vi "Data Stream Control.vi"(4 "ready for input?":bool=TRUE caption="ready for input? (true)", 6 "force error":bool caption="force error (false)", 7 "stream.num samples 0":u64, 9 "data valid":bool=TRUE caption="data valid (true)", 10 "element count":u16=1 caption="element count (1)", 11 "stream.request state 0":T1) -> (0 "request data":bool, 1 "send data":bool, 2 "stream.state 0":T1, 3 "stream.samples transferred 0":u64, 5 "stream.metadata 0":u64)   [LabVIEW 2015, in "niInstr Streaming v1 FPGA.lvlib"]
doc: "<B>General</B>\n\nThis VI gates the assertion of <B>send data</B> with a state machine controller. This enables the control and monitoring of finite and continuous streams of data.\n\n<B>Signals</B>\n\nThe stream is controlled by the <B>stream.request state</B> and <B>stream.num samples</B> inputs. The stream is monitored by the <B>stream.state</B> and <B>stream.samples transferred</B> outputs. In addition, <b>stream.metadata</b> is available for publishing details about the form/function of the stream.\n\nWhen <B>data valid</B> is True, and <B>ready for input?</B> is True, the Data Stream Control will assert <B>send data</B> until the transfer completes.\n\nWhen <B>data valid</B> is True, but <B>ready for input?</B> is False, the stream stops asserting <B>send data</B> and enters the \"Error\" state.\n\nWhen <B>force error</B> is True, the stream is forced into the Error state. This allows user logic to monitor for fatal conditions and stop the stream.\n\n<B>stream.samples transferred</B> is updated after the \"data valid\" clock cycle that increments it. This enables this output to have an easier time meeting the timed loop deadline, as well as enables it to be directly wired up as an indexing input to a write memory element.\n\n<B>request data</b> informs upstream nodes that the Data Stream Control is requesting data delivery in the next clock cycle.\n\nNote, however, that the Data Stream Control does not provide caching. Typical users wishing to avoid overflows should directly connect the \"ready for input?\" terminal to upstream data, as well as to the Data Stream Control.\n\n<b>ready for data?</b> informs the Data Stream Control that the downstream node is ready to accept data.\n\n<B>Detailed Operation</B>\n\nThe state machine has two fundamental modes of transfer: \"Finite\" and \"Continuous.\"\n\nIn Finite mode, the state machine will count <B>stream.num samples</B> in increments of <B>element count</B>. When the count is equal to or exceeds <B>stream.num samples</B>, it prevents the assertion of <B>send data</B> and enters the Done state. In the \"Done\" state the samples transferred continues to be reported until the user requests that the state machine return to \"Idle.\"\n\nIn Continuous mode, the state machine will behave identically to Finite mode, but will continously transfer samples instead of counting them.\n\n<b>States</b>\n\nThere are seven potential states for a stream defined by the Stream State.ctl typedef. All commanded states should be monitored from the controlling loop if it is important to ensure that the state is actually entered. The <B>stream.request state</B> commands the stream into a state, and <B>stream.state</B> reflects the current actual state.\n\n\nIdle - when the stream is ready to enter into an active state, it is in the Idle state. While it can be commanded directly to Idle from any state (other than Not Ready), it is advisable to do so with caution as samples abandoned in transfers may still need to be manually cleared out. It is generally safe to go directly from \"Done\" to \"Idle,\" and it is generally safe to request a transition from \"Not Ready\" to \"Idle.\" Other states may require further clean-up such as stopping/starting FIFOs or resetting other code under the command of the stream. Consider using \"Cancel\" instead (such as through the \"Stop Stream.vi\" in the host environment).\n\nWhile in Idle, <B>stream.samples transferred</B> is reset to 0. \n\nFinite Transfer - Execute a transfer for the requested number of samples. <B>data valid</B> is passed through to <B>send data</B> until the stream terminates. Upon an orderly completion, this VI will automatically enter the Done state. If a stream overflows because <B>data valid</B> is True, but <B>ready for input?</B> is False, the stream stops asserting <B>send data</B> and enters the \"Error\" state.\n\nContinuous - Execute a transfer indefinitely. This state operates identically to the Finite Transfer state, but without regard to the <B>stream.num samples</B> input.\n\nDone - In an orderly termination of a finite stream, the stream should end up here. At this point, <B>stream.samples transferred</B> accurately reflects the terminal state of the transfer. The \"Done\" state should be exited by requesting \"Idle.\" \"Cancel\" or further active transfer modes (Finite or Continuous) will be ignored. This allows the host to distinguish between streams that are prematurely terminated (thus potentially requiring a flush of abandoned data) and ones that completed naturally.\n\nError - If the stream detects an unplanned interruption of the data, it enters the Error state. The error state is normally considered a fatal state, although one may enter it purposefully (such as at the end of a long, Continuous mode Host to Target transfer). The only way to exit the Error state is to command the Data Stream Control back to Idle, or reset the FPGA VI. When commanded to Idle, the Data Stream Control advances first to \"Not Ready.\" See that state for more information.\n\nNot Ready - In this state, the FPGA remains Not Ready until the \"ready for input?\" parameter becomes true. This prevents starting a transfer in an obviously invalid state, and allows host control to wait until the \"not ready\" state is removed (such as by clearing out a FIFO under the streaming API's control). Although unusual to command the stream into this state, a client may use the features of this state to avoid going to idle until the FPGA indicates readiness.\n\nCancel - this state is indistinguishable from \"Done,\" but allows the controlling VI to know what condition caused the transfer to terminate."
uses:
  <instrlib>/_niInstr/Streaming/v1/FPGA/niInstr Streaming v1 FPGA.lvlib
  <instrlib>/_niInstr/Streaming/v1/Common/Stream State.ctl
  <instrlib>/_niInstr/Streaming/v1/Common/niInstr Streaming v1 Common.lvlib
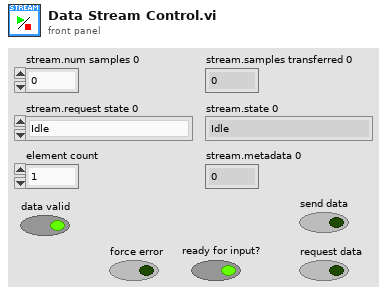
[diagram p1: front panel]
types:
  T1 = typedef "niInstr Streaming v1 Common.lvlib/Stream State.ctl" = enum8{"Idle", "Finite Transfer", "Continuous", "Done", "Error", "Not Ready", "Cancel"}
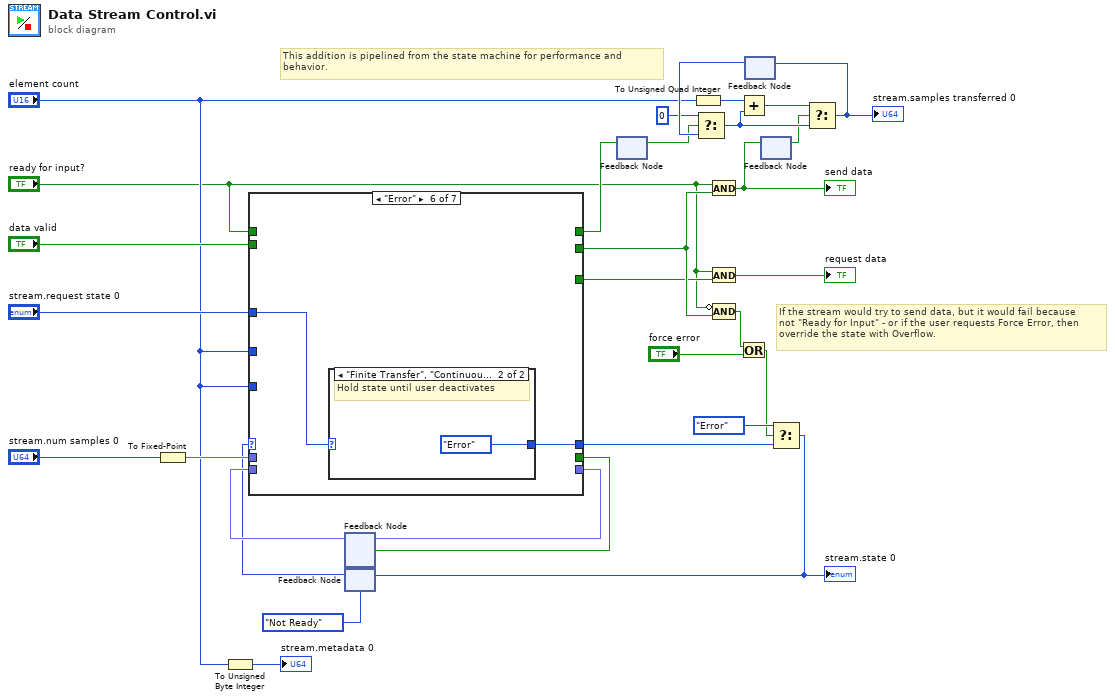
[diagram p0: block diagram]
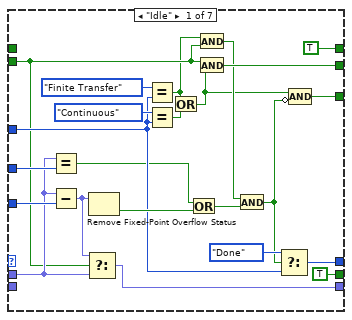
[diagram p2: hidden frame]
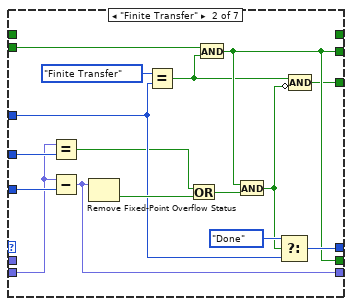
[diagram p3: hidden frame]
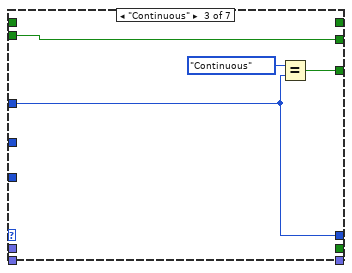
[diagram p4: hidden frame]
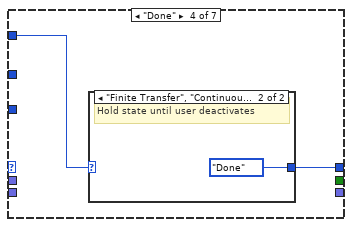
[diagram p5: hidden frame]
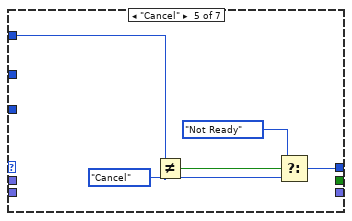
[diagram p7: hidden frame]
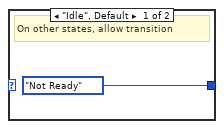
[diagram p8: hidden frame]
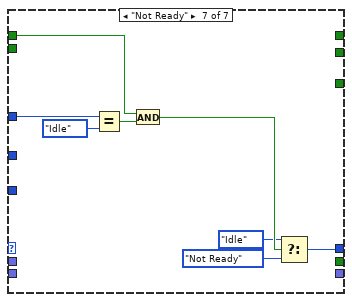
[diagram p9: hidden frame]
diagram:
  # "If the stream would try to send data, but it would fail because\nnot \"Ready for Input\" - or if the user requests Force Error, then\noverride the state with Overflow."
  # "This addition is pipelined from the state machine for performance and behavior."
  n1 = To Fixed-Point(number="stream.num samples 0") -> (fixed-point=w18:fxp<+,48,48>)  [unwired: 1 in]
  n2 = To Unsigned Byte Integer(number="element count") -> (unsigned 8bit integer=→"stream.metadata 0":u8)
  n3 = feedback #1() -> (w16:fxp<+,48,48>)  [unwired: 1 in]
  n4 = feedback #2(Stream_State."Not Ready" ("stream.state 0")) -> (w5:T1)
  n5 = case shown="\"Error\"" w5 {
    tunnel: [w49 w63 w72 w75 w83 w84 w95] -> w26
    tunnel: "stream.request state 0" -> [w44 w64 w72 w76 w81 w85 w94]
    tunnel: "data valid" -> [w37 w69 w74 _ _ _ _]
    tunnel: [w50 w58 w74 _ _ _ _] -> w25
    tunnel: [TRUE _ _ _ _ _ _] -> w11
    tunnel: w18 -> [w39 _ _ _ _ _ _]
    tunnel: "element count" -> [w53 w68 _ _ _ _ _]
    tunnel: [w38 w67 _ _ _ _ _] -> w17
    tunnel: w16 -> [_ w60 _ _ _ _ _]
    tunnel: "ready for input?" -> [_ _ _ _ _ _ w91]
    tunnel: "element count" -> [w43 w61 _ _ _ _ _]
    tunnel: [TRUE w58 _ _ _ _ _] -> w14
    tunnel: [w32 w55 w71 _ _ _ _] -> w2
    frame "Idle" {
      n6 = Equal?(x=w39, y=w43) -> (x = y?=w42:bool)
      n7 = Subtract(x=w39, y=w53) -> (x-y=w40:fxp<+,48,48>)
      n8 = Select(t=w40, s=w37, f=w39) -> (s? t:f=w38:fxp<+,48,48>)
      n9 = Remove Fixed-Point Overflow Status(3:w40) -> (0:w52:bool)  [unwired: 1 out]
      n10 = Equal?(x=Stream_State."Finite Transfer", y=w44) -> (x = y?=w36:bool)
      n11 = Equal?(x=Stream_State."Continuous", y=w44) -> (x = y?=w45:bool)
      n12 = Or(x=w36, y=w45) -> (x .or. y?=w33:bool)
      n13 = Or(x=w42, y=w52) -> (x .or. y?=w51:bool)
      n14 = And(x=w36, y=w37) -> (x .and. y?=w35:bool)
      n15 = And(x=w37, y=w33) -> (x .and. y?=w50:bool)
      n16 = And(x=w35, y=w51) -> (x .and. y?=w34:bool)
      n17 = Select(t=Stream_State."Done", s=w34, f=w44) -> (s? t:f=w49:T1)
      n18 = Compound Arithmetic op=AND(w33, invert w34) -> (w32:bool)
    }
    frame "Finite Transfer" {
      n19 = Equal?(x=w60, y=w61) -> (x = y?=w59:bool)
      n20 = Subtract(x=w60, y=w68) -> (x-y=w67:fxp<+,48,48>)
      n21 = Remove Fixed-Point Overflow Status(3:w67) -> (0:w66:bool)  [unwired: 1 out]
      n22 = Equal?(x=Stream_State."Finite Transfer", y=w64) -> (x = y?=w56:bool)
      n23 = Or(x=w59, y=w66) -> (x .or. y?=w65:bool)
      n24 = And(x=w69, y=w56) -> (x .and. y?=w58:bool)
      n25 = And(x=w58, y=w65) -> (x .and. y?=w57:bool)
      n26 = Select(t=Stream_State."Done", s=w57, f=w64) -> (s? t:f=w63:T1)
      n27 = Compound Arithmetic op=AND(w56, invert w57) -> (w55:bool)
    }
    frame "Continuous" {
      n28 = Equal?(x=Stream_State."Continuous", y=w72) -> (x = y?=w71:bool)
    }
    frame "Done" {
      n29 = case shown="\"Finite Transfer\", \"Continuous\"" w76 {
        selector: w76 -> [w77 _]
        tunnel: [w77 Stream_State."Done" ("stream.state 0")] -> w75
        frame "Idle", Default {
          # "On other states, allow transition"
        }
        frame "Finite Transfer", "Continuous" {
          # "Hold state until user deactivates"
        }
      }
    }
    frame "Cancel" {
      w82 = Stream_State."Cancel" ("stream.request state 0")
      n30 = Not Equal?(x=w81, y=w82) -> (x != y?=w80:bool)
      n31 = Select(t=Stream_State."Not Ready" ("stream.request state 0"), s=w80, f=w82) -> (s? t:f=w83:T1)
    }
    frame "Error" {
      n32 = case shown="\"Finite Transfer\", \"Continuous\", \"Error\", \"Cancel\"" w85 {
        tunnel: [Stream_State."Not Ready" ("f") Stream_State."Error" ("stream.state 0")] -> w84
        frame "Idle", Default {
          # "On other states, allow transition"
        }
        frame "Finite Transfer", "Continuous", "Error", "Cancel" {
          # "Hold state until user deactivates"
        }
      }
    }
    frame "Not Ready" {
      n33 = Equal?(x=w94, y=Stream_State."Idle" ("stream.state 0")) -> (x = y?=w92:bool)
      n34 = And(x=w91, y=w92) -> (x .and. y?=w90:bool)
      n35 = Select(t=Stream_State."Idle" ("stream.state 0"), s=w90, f=Stream_State."Not Ready" ("stream.state 0")) -> (s? t:f=w95:T1)
    }
  }
  n36 = feedback-in #1(w17, w14) -> ()
  n37 = feedback #3() -> (w10:bool)  [unwired: 1 in]
  n38 = feedback-in #3(w11) -> ()
  n39 = To Unsigned Quad Integer(1:"element count") -> (0:w7:u64)
  n40 = And(x="ready for input?", y=w25) -> (x .and. y?=w8:bool)
  "send data" <- w8
  n41 = And(x="ready for input?", y=w2) -> (x .and. y?=→"request data":bool)
  n42 = Compound Arithmetic op=AND(invert "ready for input?", w25) -> (w30:bool)
  n43 = Or(x=w30, y="force error") -> (x .or. y?=w13:bool)
  n44 = feedback #4() -> (w21:u64)  [unwired: 1 in]
  n45 = Select(t=u64 0 ("f"), s=w10, f=w21) -> (s? t:f=w22:u64)
  n46 = Add(x=w7, y=w22) -> (x+y=w24:u64)
  n47 = feedback #5() -> (w9:bool)  [unwired: 1 in]
  n48 = feedback-in #5(w8) -> ()
  n49 = Select(t=Stream_State."Error", s=w13, f=w26) -> (s? t:f=w28:T1)
  "stream.state 0" <- w28
  n50 = feedback-in #2(w28) -> ()
  n51 = Select(t=w24, s=w9, f=w22) -> (s? t:f=w23:u64)
  "stream.samples transferred 0" <- w23
  n52 = feedback-in #4(w23) -> ()
